vi "Periodic Tasks.vi"(8 "error in":errorcluster, 11 "RobotConfig":T6={"Motors"={"RightDrivePrimary"={"CAN Address"=0, "Invert"=FALSE, "InvertSensor"=FALSE, "Unit Conversion Factor"=0.0, "Brake Mode"=enum."Override to Brake", "Reverse Limt Switch Mode"=enum."Disabled", "Forward Limt Swith Mode"=enum."Disabled", "PWM Channel"=enum."Invalid", "Motor Controller Type"=enum."Talon SRX", "Peak Current (A)"=0, "Continuous Current (A)"=0, "Peak Duration (ms)"=0, "Current Limit Enable"=FALSE}, "RightDriveSecondary"={"CAN Address"=0, "Invert"=FALSE, "InvertSensor"=FALSE, "Unit Conversion Factor"=0.0, "Brake Mode"=enum."Override to Brake", "Reverse Limt Switch Mode"=enum."Disabled", "Forward Limt Swith Mode"=enum."Disabled", "PWM Channel"=enum."Invalid", "Motor Controller Type"=enum."Talon SRX", "Peak Current (A)"=0, "Continuous Current (A)"=0, "Peak Duration (ms)"=0, "Current Limit Enable"=FALSE}, "LeftDrivePrimary"={"CAN Address"=0, "Invert"=FALSE, "InvertSensor"=FALSE, "Unit Conversion Factor"=0.0, "Brake Mode"=enum."Override to Brake", "Reverse Limt Switch Mode"=enum."Disabled", "Forward Limt Swith Mode"=enum."Disabled", "PWM Channel"=enum."Invalid", "Motor Controller Type"=enum."Talon SRX", "Peak Current (A)"=0, "Continuous Current (A)"=0, "Peak Duration (ms)"=0, "Current Limit Enable"=FALSE}, "LeftDriveSecondary"={"CAN Address"=0, "Invert"=FALSE, "InvertSensor"=FALSE, "Unit Conversion Factor"=0.0, "Brake Mode"=enum."Override to Brake", "Reverse Limt Switch Mode"=enum."Disabled", "Forward Limt Swith Mode"=enum."Disabled", "PWM Channel"=enum."Invalid", "Motor Controller Type"=enum."Talon SRX", "Peak Current (A)"=0, "Continuous Current (A)"=0, "Peak Duration (ms)"=0, "Current Limit Enable"=FALSE}, "RightShooter"={"CAN Address"=0, "Invert"=FALSE, "InvertSensor"=FALSE, "Unit Conversion Factor"=0.0, "Brake Mode"=enum."Override to Brake", "Reverse Limt Switch Mode"=enum."Disabled", "Forward Limt Swith Mode"=enum."Disabled", "PWM Channel"=enum."Invalid", "Motor Controller Type"=enum."Talon SRX", "Peak Current (A)"=0, "Continuous Current (A)"=0, "Peak Duration (ms)"=0, "Current Limit Enable"=FALSE}, "LeftShooter"={"CAN Address"=0, "Invert"=FALSE, "InvertSensor"=FALSE, "Unit Conversion Factor"=0.0, "Brake Mode"=enum."Override to Brake", "Reverse Limt Switch Mode"=enum."Disabled", "Forward Limt Swith Mode"=enum."Disabled", "PWM Channel"=enum."Invalid", "Motor Controller Type"=enum."Talon SRX", "Peak Current (A)"=0, "Continuous Current (A)"=0, "Peak Duration (ms)"=0, "Current Limit Enable"=FALSE}, "ShooterRotate"={"CAN Address"=0, "Invert"=FALSE, "InvertSensor"=FALSE, "Unit Conversion Factor"=0.0, "Brake Mode"=enum."Override to Brake", "Reverse Limt Switch Mode"=enum."Disabled", "Forward Limt Swith Mode"=enum."Disabled", "PWM Channel"=enum."Invalid", "Motor Controller Type"=enum."Talon SRX", "Peak Current (A)"=0, "Continuous Current (A)"=0, "Peak Duration (ms)"=0, "Current Limit Enable"=FALSE}, "ShooterHood"={"CAN Address"=0, "Invert"=FALSE, "InvertSensor"=FALSE, "Unit Conversion Factor"=0.0, "Brake Mode"=enum."Override to Brake", "Reverse Limt Switch Mode"=enum."Disabled", "Forward Limt Swith Mode"=enum."Disabled", "PWM Channel"=enum."Invalid", "Motor Controller Type"=enum."Talon SRX", "Peak Current (A)"=0, "Continuous Current (A)"=0, "Peak Duration (ms)"=0, "Current Limit Enable"=FALSE}, "HopperWheel"={"CAN Address"=0, "Invert"=FALSE, "InvertSensor"=FALSE, "Unit Conversion Factor"=0.0, "Brake Mode"=enum."Override to Brake", "Reverse Limt Switch Mode"=enum."Disabled", "Forward Limt Swith Mode"=enum."Disabled", "PWM Channel"=enum."Invalid", "Motor Controller Type"=enum."Talon SRX", "Peak Current (A)"=0, "Continuous Current (A)"=0, "Peak Duration (ms)"=0, "Current Limit Enable"=FALSE}, "Elevator"={"CAN Address"=0, "Invert"=FALSE, "InvertSensor"=FALSE, "Unit Conversion Factor"=0.0, "Brake Mode"=enum."Override to Brake", "Reverse Limt Switch Mode"=enum."Disabled", "Forward Limt Swith Mode"=enum."Disabled", "PWM Channel"=enum."Invalid", "Motor Controller Type"=enum."Talon SRX", "Peak Current (A)"=0, "Continuous Current (A)"=0, "Peak Duration (ms)"=0, "Current Limit Enable"=FALSE}, "ClimberLeft"={"CAN Address"=0, "Invert"=FALSE, "InvertSensor"=FALSE, "Unit Conversion Factor"=0.0, "Brake Mode"=enum."Override to Brake", "Reverse Limt Switch Mode"=enum."Disabled", "Forward Limt Swith Mode"=enum."Disabled", "PWM Channel"=enum."Invalid", "Motor Controller Type"=enum."Talon SRX", "Peak Current (A)"=0, "Continuous Current (A)"=0, "Peak Duration (ms)"=0, "Current Limit Enable"=FALSE}, "ClimberRight"={"CAN Address"=0, "Invert"=FALSE, "InvertSensor"=FALSE, "Unit Conversion Factor"=0.0, "Brake Mode"=enum."Override to Brake", "Reverse Limt Switch Mode"=enum."Disabled", "Forward Limt Swith Mode"=enum."Disabled", "PWM Channel"=enum."Invalid", "Motor Controller Type"=enum."Talon SRX", "Peak Current (A)"=0, "Continuous Current (A)"=0, "Peak Duration (ms)"=0, "Current Limit Enable"=FALSE}, "Intake"={"CAN Address"=0, "Invert"=FALSE, "InvertSensor"=FALSE, "Unit Conversion Factor"=0.0, "Brake Mode"=enum."Override to Brake", "Reverse Limt Switch Mode"=enum."Disabled", "Forward Limt Swith Mode"=enum."Disabled", "PWM Channel"=enum."Invalid", "Motor Controller Type"=enum."Talon SRX", "Peak Current (A)"=0, "Continuous Current (A)"=0, "Peak Duration (ms)"=0, "Current Limit Enable"=FALSE}, "ControlPanel"={"CAN Address"=0, "Invert"=FALSE, "InvertSensor"=FALSE, "Unit Conversion Factor"=0.0, "Brake Mode"=enum."Override to Brake", "Reverse Limt Switch Mode"=enum."Disabled", "Forward Limt Swith Mode"=enum."Disabled", "PWM Channel"=enum."Invalid", "Motor Controller Type"=enum."Talon SRX", "Peak Current (A)"=0, "Continuous Current (A)"=0, "Peak Duration (ms)"=0, "Current Limit Enable"=FALSE}}, "PID"={"Shooter"={"P"=0.0, "I"=0.0, "D"=0.0, "F"=0.0, "IZone"=0.0}, "Turret"={"P"=0.0, "I"=0.0, "D"=0.0, "F"=0.0, "IZone"=0.0}, "Elevator"={"P"=0.0, "I"=0.0, "D"=0.0, "F"=0.0, "IZone"=0.0}, "ControlPanel"={"P"=0.0, "I"=0.0, "D"=0.0, "F"=0.0, "IZone"=0.0}, "Hood"={"P"=0.0, "I"=0.0, "D"=0.0, "F"=0.0, "IZone"=0.0}}, "MotionMagic"={"Turret"={"CruiseVelocity"=0, "Acceleration"=0}, "Elevator"={"CruiseVelocity"=0, "Acceleration"=0}, "ControlPanel"={"CruiseVelocity"=0, "Acceleration"=0}}, "Sensors"={"IMU"={"Yaw Axis"=enum."Z", "SPI Bus"=enum."SPI MXP", "AHRS Algorithm"=enum."Complementary", "Calibration Time (s)"=3.0, "Calibrate On Open"=TRUE}, "ElevatorBottom"={"ID"=0, "RangingMode"=enum."Short", "sampleTime(ms)"=24.0}, "ElevatorTop"={"ID"=0, "RangingMode"=enum."Short", "sampleTime(ms)"=24.0}, "ControlPanelColorSensor"={"alsIntegrationTime(ms)"=10.0, "alsGain"=40, "I2C Bus"=enum."I2C On-Board", "numProximityPulses"=5, "proximityGain"=1, "proximityLEDCurrent(mA)"=50, "proximityPulseLength(ms)"=0.01, "proximitySampleTime(ms)"=10.0}}, "Solenoids"={"Intake"={"SolenoidChannel"=enum."Solenoid 0", "Invert"=FALSE}, "ClimberRachet"={"SolenoidChannel"=enum."Solenoid 0", "Invert"=FALSE}}, "EnableCompressor"=FALSE, "RobotDimensions"={"Wheelbase(in)"=0.0, "Length(in)"=0.0}, "CameraMounting"={"LensHeight(in)"=0.0, "RotationRadius(in)"=0.0, "Pitch(deg)"=0.0}, "SensorCalibrations"={"TopToFMinBallDistance(in)"=0.0, "BottomToFMinBallDistance(in)"=0.0}, "Homing"={"Hood Homing Position (deg)"=0.0, "Turret Homing Position (deg)"=0.0}, "MotionLimits"={"Hood"={"Min (deg)"=0.0, "Max (deg)"=0.0}, "Turret"={"Min (deg)"=0.0, "Max (deg)"=0.0}}} {"Sensors"."ElevatorTop"."sampleTime(ms)" min=24.0 max=1000.0 step=1.0; "Sensors"."ElevatorBottom"."sampleTime(ms)" min=24.0 max=1000.0 step=1.0}) -> ()   [LabVIEW 2019]
doc: "This VI runs in parallel to other tasks. It can contain as many user-defined periodic loops as you need. These can carry out PID or other sorts of timed response."
uses:
  ArgosLib/ArgosLib.lvlib
  InfiniteRechargeSrc/Global_Var-RefNum/JoystickControls.vi
  InfiniteRechargeSrc/Implements/Shooter/TypeDefs/Hood_Homing_State.ctl
  InfiniteRechargeSrc/Vision/TypeDefs/VisionPipeline.ctl
  <vilib>/Playing With Fusion Inc/Playing With Fusion Lib for FRC/PWF_TMD37003_LabVIEW/PwF_TMD37003.lvlib
  <vilib>/Playing With Fusion Inc/Playing With Fusion Lib for FRC/PWF_TMD37003_LabVIEW/Public/PwF_TMD37003_RGBToHSV_SensorData.vi
  <vilib>/Rock Robotics/WPI/ThirdParty/Phoenix-LabVIEW/Motor Controller/Controls/CTRE_Phoenix_MotorControl_NeutralMode.ctl
  <vilib>/Rock Robotics/WPI/ThirdParty/Phoenix-LabVIEW/Motor Controller/Controls/CTRE_Phoenix_MotorControl_LimitSwitchNormal.ctl
  <vilib>/Rock Robotics/SystemInterfaces/DIO/FPGA_DIOPWMChannel.ctl
  ArgosLib/Config/ConfigComponents/TypeDefs/Config_MotorCtrlType.ctl
  ArgosLib/Config/ConfigComponents/TypeDefs/Config_Motor.ctl
  ArgosLib/Config/ConfigComponents/TypeDefs/Config_PIDParams.ctl
  ArgosLib/Config/ConfigComponents/TypeDefs/Config_MotionMagicParams.ctl
  <vilib>/Rock Robotics/SystemInterfaces/spilib/spi_bus.ctl
  ArgosLib/Config/ConfigComponents/TypeDefs/Config_IMU.ctl
  <vilib>/Rock Robotics/WPI/Solenoid/WPI_SolenoidChannel.ctl
  ArgosLib/Config/ConfigComponents/TypeDefs/Config_SingleSolenoid.ctl
  InfiniteRechargeSrc/TypeDefs/ConfigComponents/Config_RobotDimensions.ctl
  InfiniteRechargeSrc/TypeDefs/ConfigComponents/Config_CameraMounting.ctl
  InfiniteRechargeSrc/TypeDefs/ConfigComponents/Config_Robot.ctl
  <vilib>/Playing With Fusion Inc/Playing With Fusion Lib for FRC/PWF_ToF_LabVIEW/Public/TypeDefs/PwF_ToF_RangingMode.ctl
  <vilib>/Playing With Fusion Inc/Playing With Fusion Lib for FRC/PWF_ToF_LabVIEW/PwF_ToF.lvlib
  ArgosLib/Config/ConfigComponents/TypeDefs/Config_PwFToF.ctl
  ArgosLib/Miscellaneous/TypeDefs/LookUpTableParameters.ctl
  ArgosLib/Miscellaneous/TypeDefs/ArgoDriveJoystickMap.ctl
  InfiniteRechargeSrc/Implements/Control_Panel/TypeDefs/ControlPanelColor.ctl
  <vilib>/Playing With Fusion Inc/Playing With Fusion Lib for FRC/PWF_TMD37003_LabVIEW/Public/TypeDefs/PwF_TMD37003_Data.ctl
  <vilib>/Rock Robotics/SystemInterfaces/i2clib/i2c_bus.ctl
  ArgosLib/Config/ConfigComponents/TypeDefs/Config_PwF_TMD37003.ctl
panel:
  out "TMD37003 Data":T1
  out "Color":T2=enum."Blue"
  out "Turret Distance (in)":dbl
  out "Shooter Velocity":dbl
  in  "ManualShooterSpeed":bool
  in  "ShooterSpeed(rpm)":dbl(slide)=4000.0 min=0.0 max=10000.0 step=1.0 scale=0.0..10000.0
  in  "DisableLimelight":bool
  out "Target Found?":bool
  in  "SetPointTurret(Deg)":dbl(slide) scale=-108.0..108.0
  in  "Activate Auto (Turret)":bool
  out "TurretManual":bool
  out "Turret Current Position (Deg)":dbl
  out "Hood Current Position (Deg)":dbl
  out "HoodManual?":bool
  in  "Activate Auto (Shooter Hood)":bool
  in  "SetPointHood(Deg)":dbl
  in  "TurretHomeReset":bool
  in  "Turret Homing Activated":bool
  out "Turret Homing_State":T3
  in  "HoodHomeActivate":bool
  in  "HoodHomeReset":bool
  out "Hood_Homing_State":T3
  in  "Argo Drive Joystick Map":T4={"Auto Speed"={"Look Up Table OUT"=[-1.0, 0.0, 1.0], "Look Up Table IN"=[-1.0, 0.0, 1.0]}, "Low Speed"={"Look Up Table OUT"=[-1.0, 0.0, 0.0, 1.0], "Look Up Table IN"=[-1.0, -0.25, 0.25, 1.0]}, "Auto Turning"={"Look Up Table OUT"=[-1.0, 0.0, 1.0], "Look Up Table IN"=[-1.0, 0.0, 1.0]}, "Low Turning"={"Look Up Table OUT"=[-1.0, 0.0, 0.0, 1.0], "Look Up Table IN"=[-1.0, -0.25, 0.25, 1.0]}, "High Speed"={"Look Up Table OUT"=[], "Look Up Table IN"=[]}, "High Turning"={"Look Up Table OUT"=[], "Look Up Table IN"=[]}}
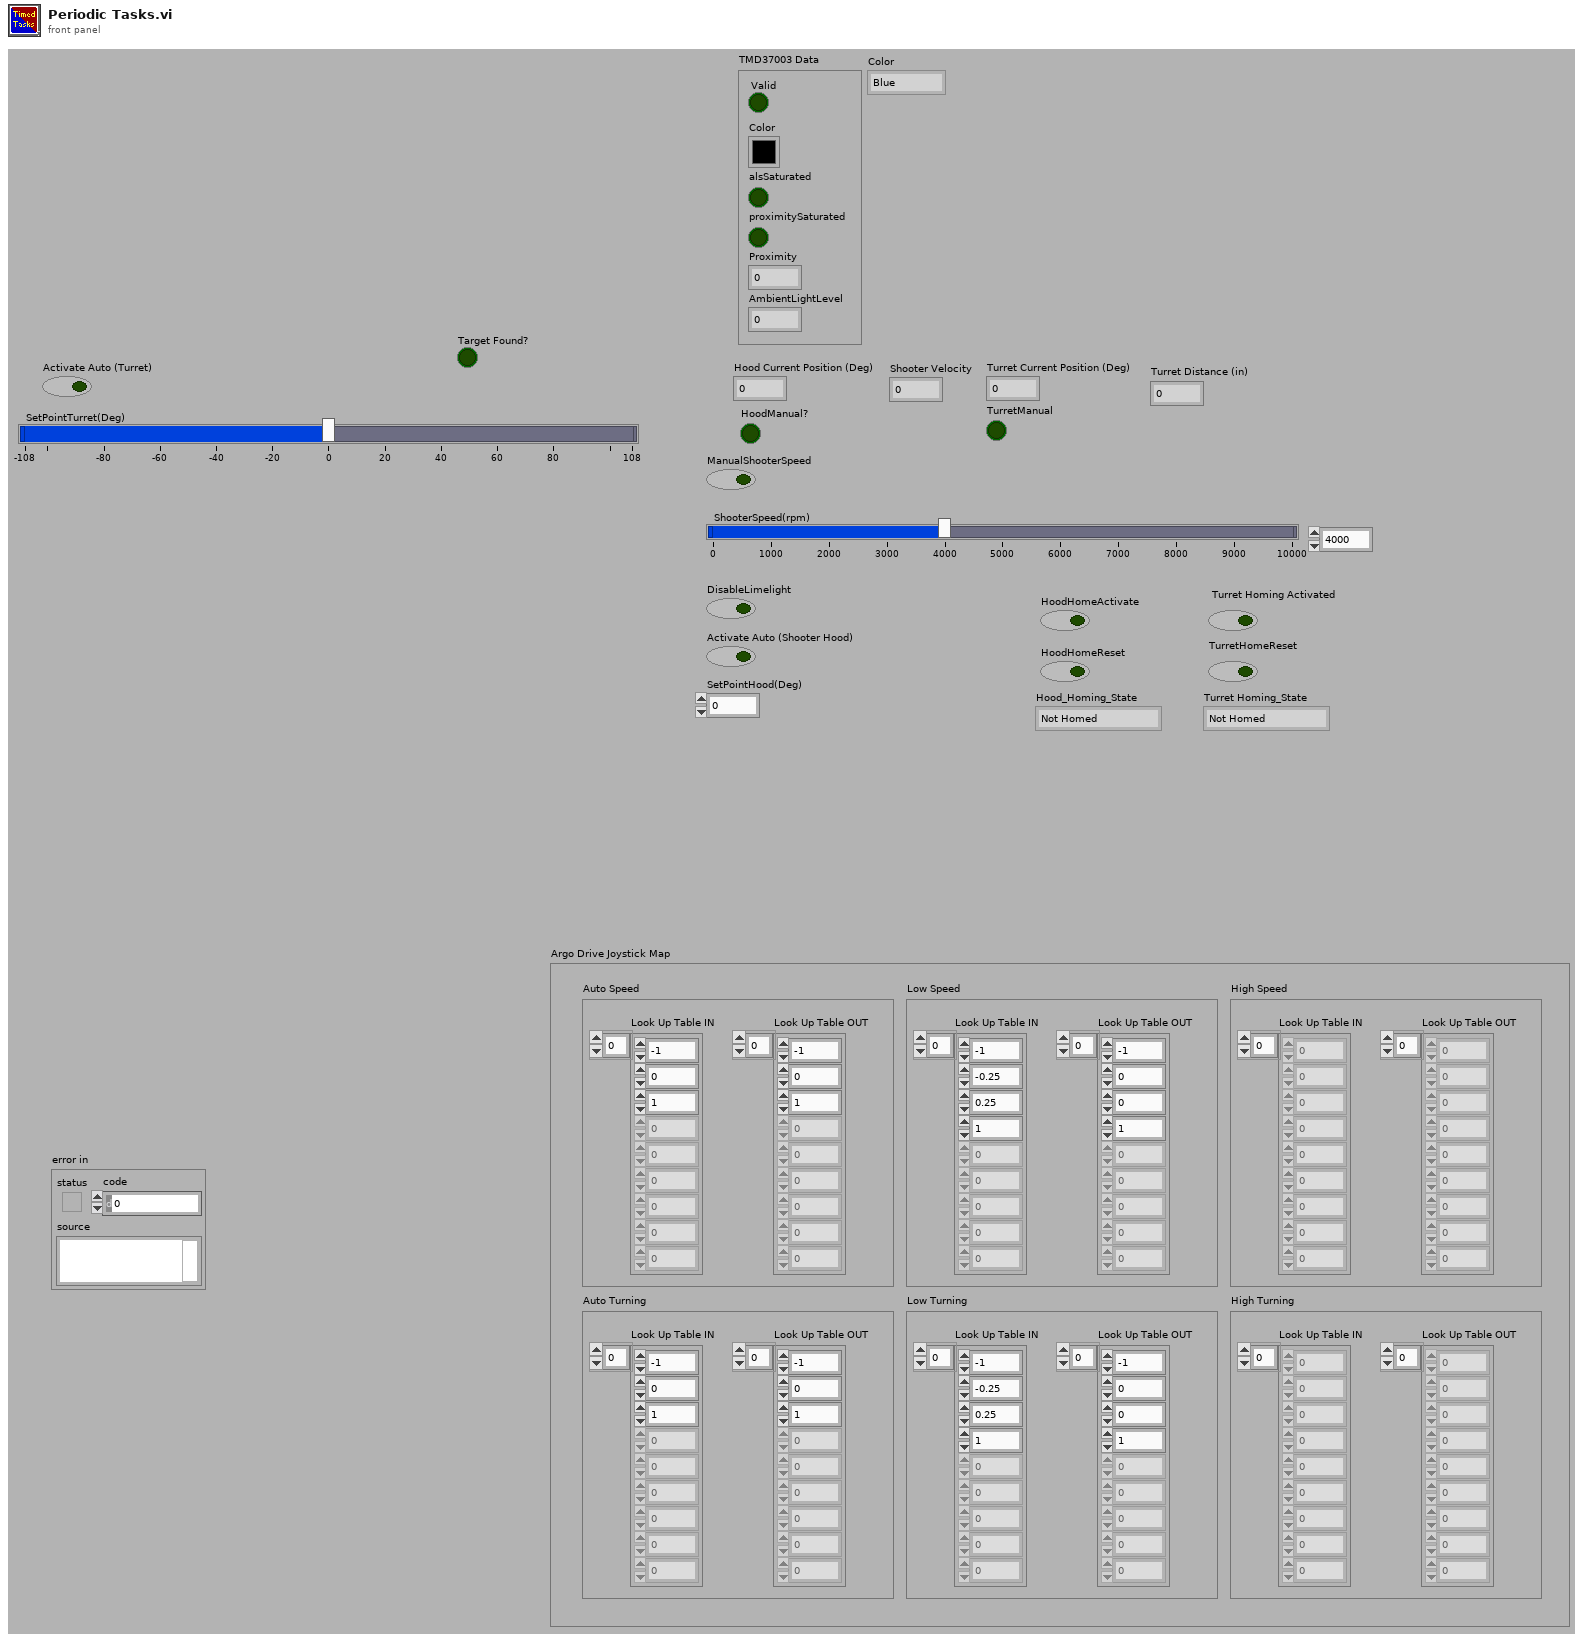
[diagram p1: front panel]
types:
  T1 = typedef "PlayingWithFusionLib.lvlib/PwF_TMD37003.lvlib/PwF_TMD37003_Data.ctl" = cluster{"Valid":bool, "Color":u32, "alsSaturated":bool, "proximitySaturated":bool, "Proximity":dbl, "AmbientLightLevel":dbl}
  T2 = typedef "ControlPanelColor.ctl" = enum16{"Unknown", "Red", "Green", "Blue", "Yellow"}
  T3 = typedef "Hood_Homing_State.ctl" = enum16{"Not Homed", "Homing in Process", "Homing Failed", "Homing Completed"}
  T4 = typedef "ArgosLib.lvlib/ArgoDriveJoystickMap.ctl" = cluster{"Auto Speed":T5, "Low Speed":T5, "Auto Turning":T5, "Low Turning":T5, "High Speed":T5, "High Turning":T5}
  T5 = typedef "ArgosLib.lvlib/LookUpTableParameters.ctl" = cluster{"Look Up Table OUT":dbl[], "Look Up Table IN":dbl[]}
  T6 = typedef "Config_Robot.ctl" = cluster{"Motors":cluster{"RightDrivePrimary":T7, "RightDriveSecondary":T7, "LeftDrivePrimary":T7, "LeftDriveSecondary":T7, "RightShooter":T7, "LeftShooter":T7, "ShooterRotate":T7, "ShooterHood":T7, "HopperWheel":T7, "Elevator":T7, "ClimberLeft":T7, "ClimberRight":T7, "Intake":T7, "ControlPanel":T7}, "PID":cluster{"Shooter":T12, "Turret":T12, "Elevator":T12, "ControlPanel":T12, "Hood":T12}, "MotionMagic":cluster{"Turret":T13, "Elevator":T13, "ControlPanel":T13}, "Sensors":cluster{"IMU":T14, "ElevatorBottom":T16, "ElevatorTop":T16, "ControlPanelColorSensor":T18}, "Solenoids":cluster{"Intake":T20, "ClimberRachet":T20}, "EnableCompressor":bool, "RobotDimensions":T22, "CameraMounting":T23, "SensorCalibrations":cluster{"TopToFMinBallDistance(in)":dbl, "BottomToFMinBallDistance(in)":dbl}, "Homing":cluster{"Hood Homing Position (deg)":dbl, "Turret Homing Position (deg)":dbl}, "MotionLimits":cluster{"Hood":cluster{"Min (deg)":dbl, "Max (deg)":dbl}, "Turret":cluster{"Min (deg)":dbl, "Max (deg)":dbl}}}
  T7 = typedef "ArgosLib.lvlib/Config_Motor.ctl" = cluster{"CAN Address":u8, "Invert":bool, "InvertSensor":bool, "Unit Conversion Factor":dbl, "Brake Mode":T8, "Reverse Limt Switch Mode":T9, "Forward Limt Swith Mode":T9, "PWM Channel":T10, "Motor Controller Type":T11, "Peak Current (A)":i32, "Continuous Current (A)":i32, "Peak Duration (ms)":i32, "Current Limit Enable":bool}
  T8 = typedef "CTRE_Phoenix_MotorControl_NeutralMode.ctl" = enum8{"EEPROMSetting", "Override to Coast", "Override to Brake"}
  T9 = typedef "CTRE_Phoenix_MotorControl_LimitSwitchNormal.ctl" = enum16{"Normally Open", "Normally Closed", "Disabled"}
  T10 = typedef "FPGA_DIOPWMChannel.ctl" = enum8{"PWM 0", "PWM 1", "PWM 2", "PWM 3", "PWM 4", "PWM 5", "PWM 6", "PWM 7", "PWM 8", "PWM 9", "PWM MXP 0", "PWM MXP 1", "PWM MXP 2", "PWM MXP 3", "PWM MXP 4", "PWM MXP 5", "PWM MXP 6", "PWM MXP 7", "PWM MXP 8", "PWM MXP 9", "Invalid"}
  T11 = typedef "ArgosLib.lvlib/Config_MotorCtrlType.ctl" = enum16{"Disabled", "Talon SRX", "Talon SR", "Venom", "Spark MAX", "Falcon FX"}
  T12 = typedef "ArgosLib.lvlib/Config_PIDParams.ctl" = cluster{"P":dbl, "I":dbl, "D":dbl, "F":dbl, "IZone":dbl}
  T13 = typedef "ArgosLib.lvlib/Config_MotionMagicParams.ctl" = cluster{"CruiseVelocity":i32, "Acceleration":i32}
  T14 = typedef "ArgosLib.lvlib/Config_IMU.ctl" = cluster{"Yaw Axis":enum16{"X", "Y", "Z"}, "SPI Bus":T15, "AHRS Algorithm":enum16{"Complementary", "Madgwick"}, "Calibration Time (s)":dbl, "Calibrate On Open":bool}
  T15 = typedef "spi_bus.ctl" = enum16{"SPI On-Board, CS0", "SPI On-Board, CS1", "SPI On-Board, CS2", "SPI On-Board, CS3", "SPI MXP", "Invalid"}
  T16 = typedef "ArgosLib.lvlib/Config_PwFToF.ctl" = cluster{"ID":u8, "RangingMode":T17, "sampleTime(ms)":dbl}
  T17 = typedef "PlayingWithFusionLib.lvlib/PwF_ToF.lvlib/PwF_ToF_RangingMode.ctl" = enum16{"Short", "Medium", "Long"}
  T18 = typedef "ArgosLib.lvlib/Config_PwF_TMD37003.ctl" = cluster{"alsIntegrationTime(ms)":dbl, "alsGain":u8, "I2C Bus":T19, "numProximityPulses":u8, "proximityGain":u8, "proximityLEDCurrent(mA)":u8, "proximityPulseLength(ms)":dbl, "proximitySampleTime(ms)":dbl}
  T19 = typedef "i2c_bus.ctl" = enum16{"I2C On-Board", "I2C MXP", "Invalid"}
  T20 = typedef "ArgosLib.lvlib/Config_SingleSolenoid.ctl" = cluster{"SolenoidChannel":T21, "Invert":bool}
  T21 = typedef "WPI_SolenoidChannel.ctl" = enum8{"Solenoid 0", "Solenoid 1", "Solenoid 2", "Solenoid 3", "Solenoid 4", "Solenoid 5", "Solenoid 6", "Solenoid 7", "Invalid"}
  T22 = typedef "Config_RobotDimensions.ctl" = cluster{"Wheelbase(in)":dbl, "Length(in)":dbl}
  T23 = typedef "Config_CameraMounting.ctl" = cluster{"LensHeight(in)":dbl, "RotationRadius(in)":dbl, "Pitch(deg)":dbl}
  T24 = typedef "SensorRefNums.ctl" = cluster{"ElevatorBottom":T25, "ElevatorTop":T25, "ControlPanelColor":T26}
  T25 = typedef "PlayingWithFusionLib.lvlib/PwF_ToF.lvlib/PwF_ToF_DevRef.ctl" = cluster{"DeviceStatus":errorcluster, "Device Number":u8, "Handle":u64, "Library Path":path}
  T26 = typedef "PlayingWithFusionLib.lvlib/PwF_TMD37003.lvlib/PwF_TMD37003_DevRef.ctl" = cluster{"DevStatus":errorcluster, "Device Address":u8, "Handle":i32, "I2C Bus":T19}
  T27 = typedef "JoystickRefNums.ctl" = cluster{"Joystick0":T28, "Joystick1":T28}
  T28 = typedef "WPI_JoystickDevRef.ctl" = cluster{"Device":T29}
  T29 = typedef "WPI_JoystickDeviceEnum.ctl" = enum16{"USB 0", "USB 1", "USB 2", "USB 3", "USB 4", "USB 5"}
  T30 = typedef "WPI_RobotDriveDevRef.ctl" = cluster{"DevStatus":errorcluster, "Motors[]":T31[], "Square Inputs":bool, "Max Output":dbl}
  T31 = typedef "WPI_MotorControlDeviceRef.ctl" = cluster{"DeviceStatus":errorcluster, "Type":T32, "PWM":cluster{"PWM Channel":T10, "DeadBand":T33}, "CAN":cluster{"Device Number":u8, "SetOutput VI Ref":variant, "GetOutput VI Ref":variant, "Enable VI Ref":variant, "Disable VI Ref":variant, "Data":variant}, "Invert":bool, "DIO PWM":cluster{"PWM \"Enable\" Channel":T10, "DIOChannel":T34, "PWM Rate":dbl}}
  T32 = typedef "WPI_MotorControlType.ctl" = enum16{"PWM", "CAN", "DIO PWM"}
  T33 = typedef "WPI_PWMDeadband.ctl" = cluster{"Name":string, "maxPositivePwm":i32, "minPositivePwm":i32, "centerPwm":i32, "maxNegativePwm":i32, "minNegativePwm":i32, "angularRange":u16}
  T34 = typedef "FPGA_DIOChannel.ctl" = enum8{"DIO 0", "DIO 1", "DIO 2", "DIO 3", "DIO 4", "DIO 5", "DIO 6", "DIO 7", "DIO 8", "DIO 9", "DIO MXP 0", "DIO MXP 1", "DIO MXP 2", "DIO MXP 3", "DIO MXP 4", "DIO MXP 5", "DIO MXP 6", "DIO MXP 7", "DIO MXP 8", "DIO MXP 9", "DIO MXP 10", "DIO MXP 11", "DIO MXP 12", "DIO MXP 13", "DIO MXP 14", "DIO MXP 15", "SPI Port CS1", "SPI Port CS2", "SPI Port CS3", "SPI Port MISO", "SPI Port MOSI", "Invalid"}
  T35 = typedef "PneumaticsRefNums.ctl" = cluster{"Intake":T36, "Compressor":T37, "ClimberRatchet":T36}
  T36 = typedef "WPI_SolenoidDevRef.ctl" = cluster{"DevStatus":errorcluster, "Pneumatics Control Module":u8, "Forward Solenoid Channel":T21, "Reverse Solenoid Channel":T21}
  T37 = typedef "WPI_CompressorDevRef.ctl" = cluster{"DevStatus":errorcluster, "Pneumatics Control Module":u8}
  T38 = typedef "MotorRefNums.ctl" = cluster{"LeftDrivePrimary":T31, "RightDrivePrimary":T31, "LeftDriveSecondary":T31, "RightDriveSecondary":T31, "RightShooter":T31, "LeftShooter":T31, "ShooterRotate":T31, "ShooterHood":T31, "HopperWheel":T31, "Elevator":T31, "ClimberLeft":T31, "ClimberRight":T31, "Intake":T31, "ControlPanel":T31}
  T39 = cluster{"RobotConfig":T6, "JoystickRefNums":T27, "RobotDriveDevRef":T30, "MotorRefNumsOut":T38, "Pneumatics":T35, "Sensors":T24}
  T40 = typedef "JoystickControl.ctl" = cluster{"A":bool, "B":bool, "X":bool, "Y":bool, "LB":bool, "Shoot":bool, "LJ":bool, "RJ":bool, "Back":bool, "Start":bool, "Top":bool, "Right":bool, "Bottom":bool, "Left":bool, "Eject":dbl, "Intake":dbl, "LX":dbl, "Drive Y":dbl, "Drive X":dbl, "RY":dbl, "Down":bool, "Index":bool, "Aggitate":bool, "Up":bool, "Find Target":bool, "Spin up":bool, "LJ 2":bool, "RJ 2":bool, "Back 2":bool, "Start 2":bool, "Elevate":bool, "Right 2":bool, "Retract":bool, "Left 2":bool, "Control Rotate":dbl, "RT 2":dbl, "H L/R":dbl, "H U/D":dbl, "RX 2":dbl, "RY 2":dbl}
  T41 = typedef "VisionPipeline.ctl" = enum16{"LEDOff", "NoZoom", "Zoom2x", "Zoom3x"}
  T42 = typedef "VisionTarget.ctl" = cluster{"Valid":bool, "Distance(in)":dbl, "Angle(deg)":dbl, "FieldCentricAngle(deg)":dbl, "skew (deg)":dbl}
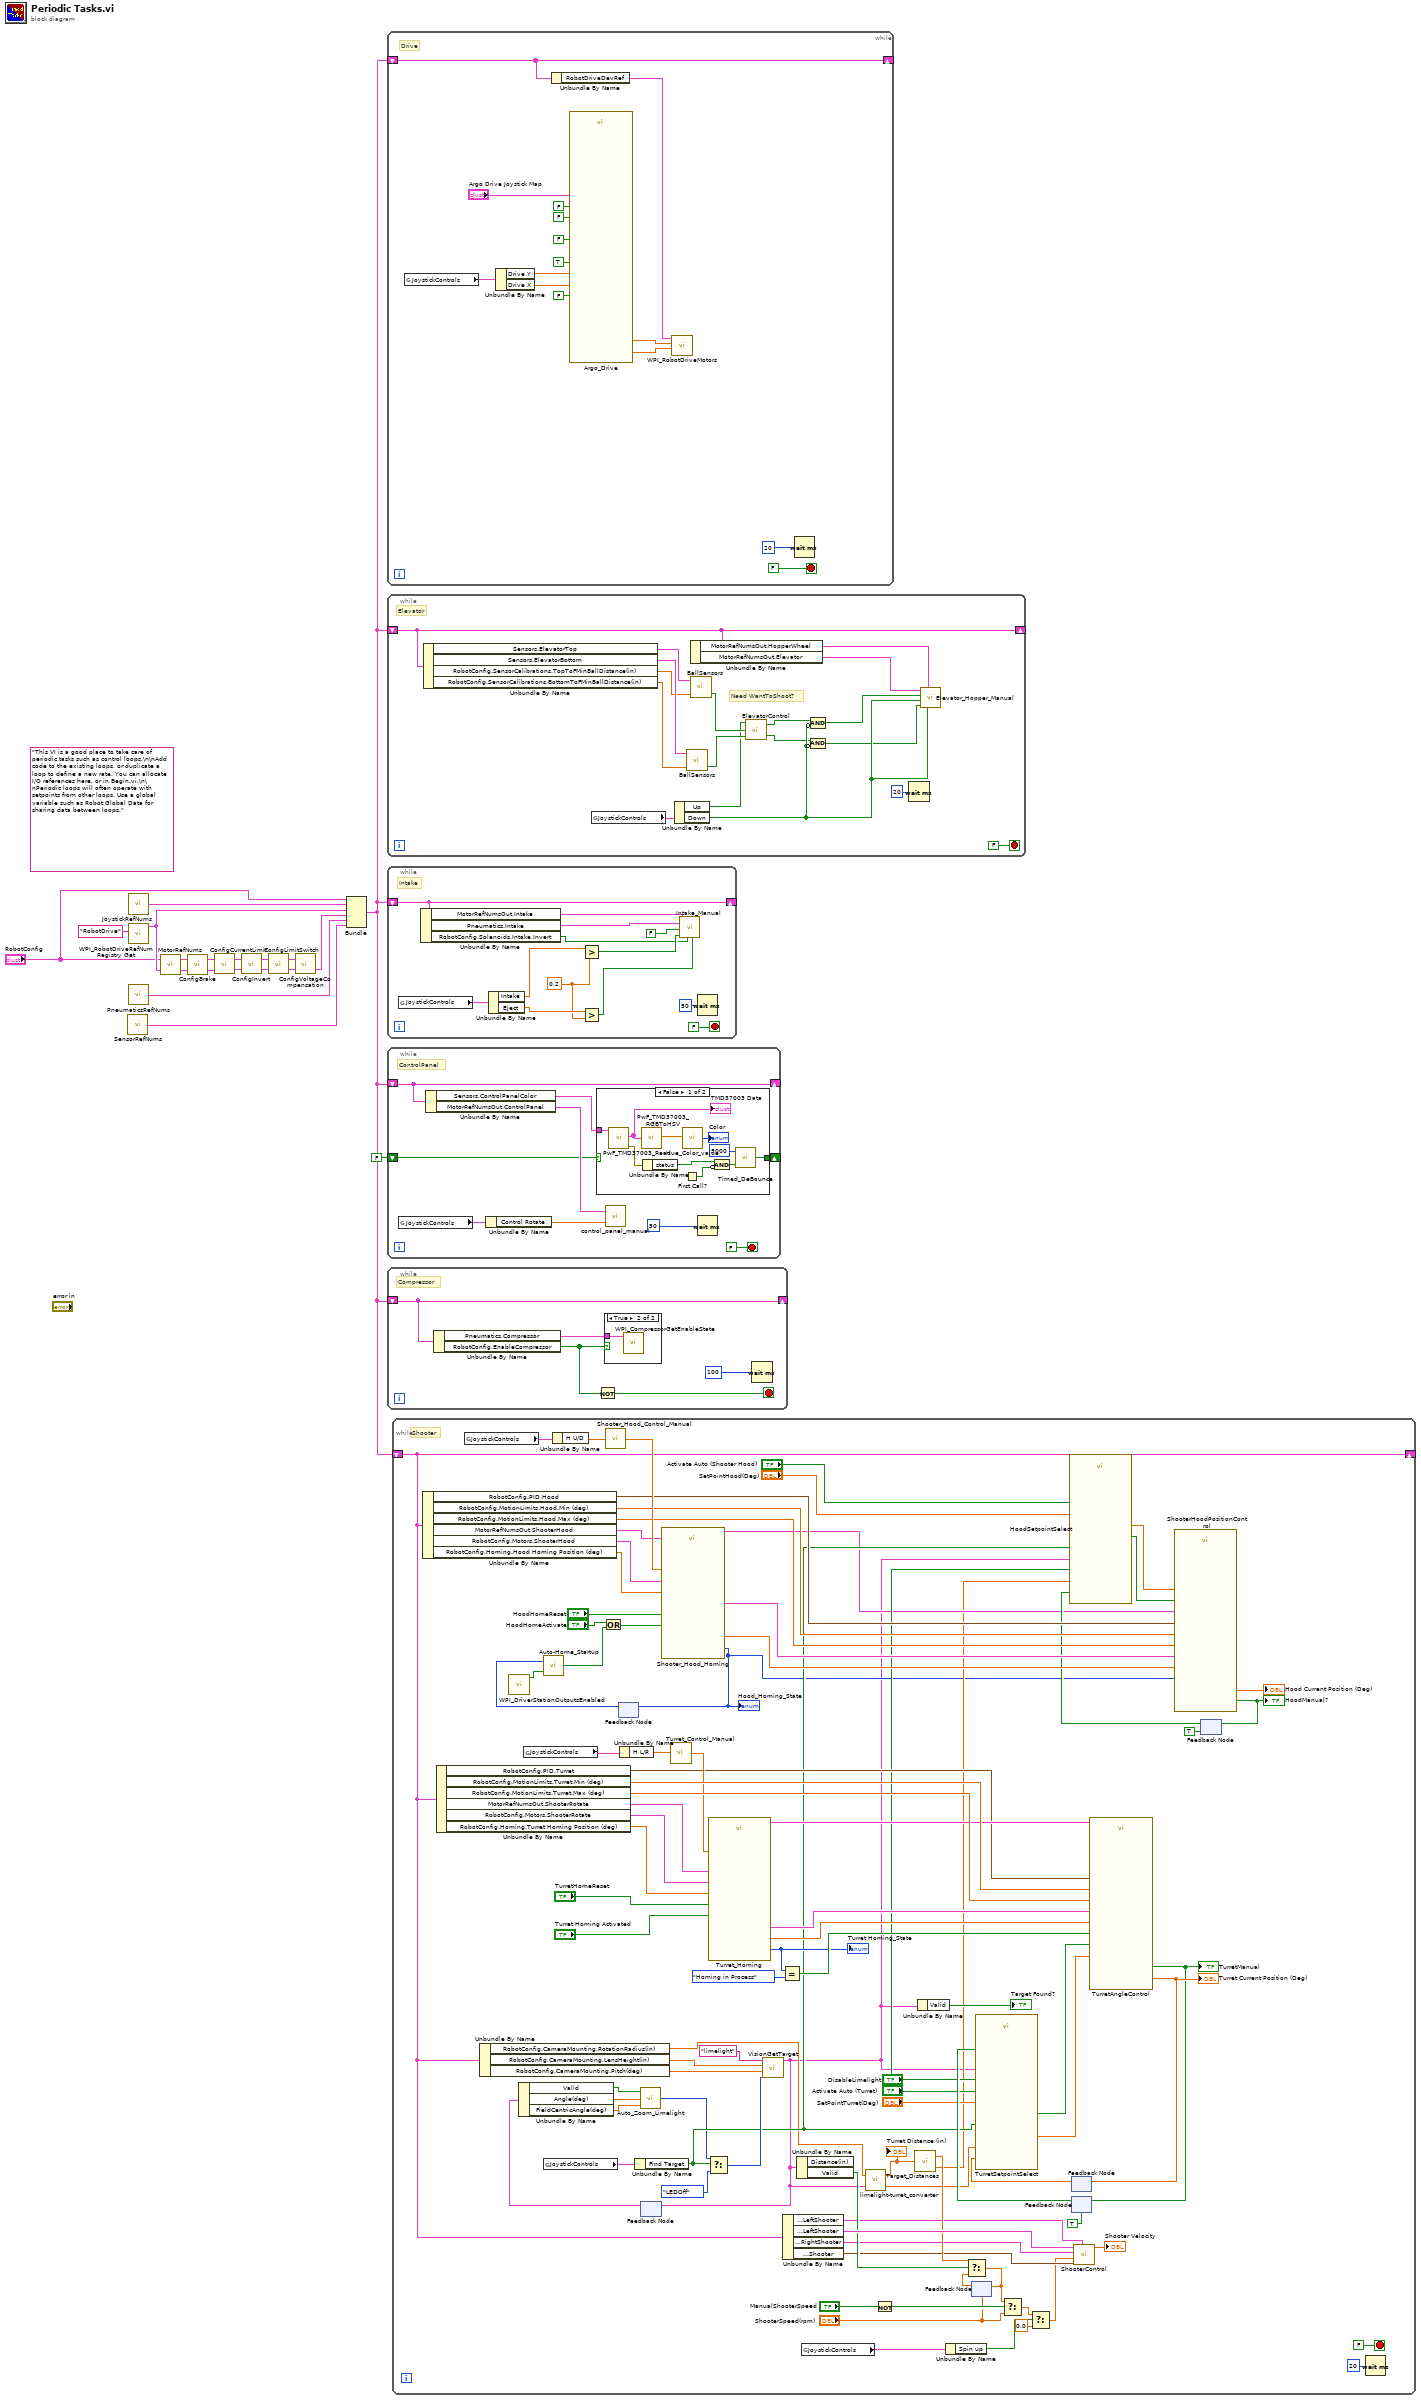
[diagram p0: block diagram]
diagram:
  (unwired) "This VI is a good place to take care of periodic tasks such as control loops.\n\nAdd code to the existing loops, or duplicate a loop to define a new rate. You can allocate I/O references here, or in Begin.vi.\n\nPeriodic loops will often operate with setpoints from other loops. Use a global variable such as Robot Global Data for sharing data between loops."
  n1 = call "SensorRefNums.vi"() -> ("Sensors"=w15:T24)  [unwired: 1 in]
  n2 = call "JoystickRefNums.vi"() -> ("JoystickRefNums"=w19:T27)  [unwired: 1 in]
  n3 = call <vilib>:"WPI_RobotDriveRefNum Registry Get.vi"("refnum name"="RobotDrive") -> ("RobotDriveDevRef"=w17:T30)  [unwired: 9 in, 1 out]
  n4 = call "PneumaticsRefNums.vi"() -> ("Pneumatics"=w16:T35)  [unwired: 1 in]
  n5 = call "MotorRefNums.vi"("RobotDriveDevRef"=w17, "RobotConfig"="RobotConfig") -> ("MotorRefNums"=w13:T38, "RobotConfigOut"=w14:T6)
  n6 = call "ConfigBrake.vi"("MotorRefNumsIn"=w13, "RobotConfigIn"=w14) -> ("MotorRefNumsOut"=w12:T38, "RobotConfigOut"=w11:T6)
  n7 = call "ConfigCurrentLimit.vi"("MotorRefNumsIn"=w12, "RobotConfigIn"=w11) -> ("MotorRefNumsOut"=w10:T38, "RobotConfigOut"=w9:T6)
  n8 = call "ConfigInvert.vi"("MotorRefNumsIn"=w10, "RobotConfigIn"=w9) -> ("MotorRefNumsOut"=w8:T38, "RobotConfigOut"=w7:T6)
  n9 = call "ConfigLimitSwitch.vi"("MotorRefNumsIn"=w8, "RobotConfigIn"=w7) -> ("MotorRefNumsOut"=w6:T38, "RobotConfigOut"=w5:T6)
  n10 = call "ConfigVoltageCompensation.vi"("MotorRefNumsIn"=w6, "RobotConfigIn"=w5) -> ("MotorRefNumsOut"=w4:T38)  [unwired: 1 out]
  n11 = Bundle("RobotConfig"="RobotConfig", "JoystickRefNums"=w19, "RobotDriveDevRef"=w17, "MotorRefNumsOut"=w4, "Pneumatics"=w16, "Sensors"=w15) -> (w2:T39)  [unwired: 1 out]
  n12 = while {
    shift-right: [w32] -> _
    shift-left: w2 -> [w32]
    stop <- FALSE stop-if-true
    # "Drive"
    n13 = global read "JoystickControls.vi" "JoystickControls"() -> (w31:T40)
    n14 = Unbundle By Name(w31) -> ("Drive Y"=w30:dbl, "Drive X"=w29:dbl)
    n15 = Unbundle By Name(w32) -> ("RobotDriveDevRef"=w22:T30)
    n16 = call "Argo_Drive.vi"("Speed_Main"=w30, "Argo Drive Joystick Map"="Argo Drive Joystick Map", "Backwards_Turning_Flip"=FALSE, "Turning_PID_Enable"=FALSE, "Turning_Main"=w29, "Auto_Enable"=FALSE, "High_Gear"=FALSE, "Quick_Turn"=TRUE) -> ("Left_Motor"=w21:dbl, "Right_Motor"=w20:dbl)  [unwired: 10 in]
    n17 = call <vilib>:"WPI_RobotDriveMotors.vi"("RightSpeed"=w20, "LeftSpeed"=w21, "RobotDriveDevRef"=w22) -> ()  [unwired: 6 in, 3 out]
    n18 = Wait (ms)(milliseconds to wait=u32 20) -> ()  [unwired: 1 out]
  }
  n19 = while {
    shift-right: [w46] -> _
    shift-left: w2 -> [w46]
    stop <- FALSE stop-if-true
    # "Need WantToShoot?"
    # "Elevator"
    n20 = Unbundle By Name(w46) -> ("Sensors.ElevatorTop"=w48:T25, "Sensors.ElevatorBottom"=w47:T25, "RobotConfig.SensorCalibrations.TopToFMinBallDistance(in)"=w38:dbl, "RobotConfig.SensorCalibrations.BottomToFMinBallDistance(in)"=w37:dbl)
    n21 = global read "JoystickControls.vi" "JoystickControls"() -> (w45:T40)
    n22 = Unbundle By Name(w45) -> ("Up"=w39:bool, "Down"=w44:bool)
    n23 = call "BallSensors.vi"("MinDistance(in.)"=w37, "BallSensorDevRefIn"=w47) -> ("BallThere?"=w50:bool)  [unwired: 1 in, 2 out]
    n24 = Unbundle By Name(w46) -> ("MotorRefNumsOut.HopperWheel"=w35:T31, "MotorRefNumsOut.Elevator"=w36:T31)
    n25 = call "BallSensors.vi"("MinDistance(in.)"=w38, "BallSensorDevRefIn"=w48) -> ("BallThere?"=w49:bool)  [unwired: 1 in, 2 out]
    n26 = call "ElevatorControl.vi"("BallThereAtBottom?"=w50, "BallThereAtTop?"=w49, "WantToShoot?"=w39) -> ("HopperWheelsOn"=w42:bool, "ElevatorOn"=w43:bool)
    n27 = Compound Arithmetic op=AND(w43, invert w44) -> (w41:bool)
    n28 = Compound Arithmetic op=AND(w42, invert w44) -> (w40:bool)
    n29 = Wait (ms)(milliseconds to wait=u32 20) -> ()  [unwired: 1 out]
    n30 = call "Elevator_Hopper_Manual.vi"("Elevator_Control"=w36, "Hopper_Control"=w35, "Elevator_up"=w41, "Elevator_Down"=w44, "Hopper Backwards"=w44, "Hopper Forwards"=w40) -> ()  [unwired: 3 in]
  }
  n31 = while {
    shift-right: [w59] -> _
    shift-left: w2 -> [w59]
    stop <- FALSE stop-if-true
    w54 = 0.2 ("y")
    # "Intake"
    n32 = global read "JoystickControls.vi" "JoystickControls"() -> (w63:T40)
    n33 = Unbundle By Name(w59) -> ("MotorRefNumsOut.Intake"=w58:T31, "Pneumatics.Intake"=w57:T36, "RobotConfig.Solenoids.Intake.Invert"=w53:bool)
    n34 = Unbundle By Name(w63) -> ("Intake"=w56:dbl, "Eject"=w55:dbl)
    n35 = Greater?(x=w56, y=w54) -> (0:w60:bool)
    n36 = Greater?(x=w55, y=w54) -> (0:w61:bool)
    n37 = call "Intake_Manual.vi"("Reverse_Intake"=w61, "Invert Solenoid"=w53, "Intake"=w60, "Disable"=FALSE, "IntakeExtendDevRef"=w57, "Intake_Motor"=w58) -> ()  [unwired: 5 in]
    n38 = Wait (ms)(milliseconds to wait=u32 50) -> ()  [unwired: 1 out]
  }
  n39 = while {
    shift-right: [w72] -> _
    shift-left: w2 -> [w72]
    shift-right: [w68] -> _
    shift-left: FALSE ("Output") -> [w67]
    stop <- FALSE stop-if-true
    # "ControlPanel"
    n40 = global read "JoystickControls.vi" "JoystickControls"() -> (w73:T40)
    n41 = Unbundle By Name(w72) -> ("Sensors.ControlPanelColor"=w71:T26, "MotorRefNumsOut.ControlPanel"=w69:T31)
    n42 = Unbundle By Name(w73) -> ("Control Rotate"=w70:dbl)
    n43 = case shown="False" w67 {
      selector: w67 -> [_ w85]
      tunnel: w71 -> [w81 _]
      tunnel: [w78 w85] -> w68
      frame False {
        n44 = call <vilib>:"PwF_TMD37003_Read.vi"("PwF_TMD37003_DevRefIn"=w81) -> ("error out"=w80:errorcluster, "TMD37003 Data"=w84:T1)  [unwired: 8 in, 1 out]
        "TMD37003 Data" <- w84
        n45 = call-poly <vilib>:"PwF_TMD37003_RGBToHSV.vi"("TMD37003 Data In"=w84) -> ("Hue"=w83:dbl)  [unwired: 3 out]
        n46 = Unbundle By Name(w80) -> ("status"=w76:bool)
        n47 = call "Hue_Color_value.vi"("Hue"=w83) -> ("Color"=→"Color":T2)
        n48 = First Call?() -> (First Call?: T/F=w77:bool)
        n49 = Compound Arithmetic op=AND(w76, invert w77) -> (w75:bool)
        n50 = call "Timed_DeBounce.vi"("Input"=w75, "Hold Time(ms)"=u32 5000) -> ("Output"=w78:bool)  [unwired: 1 in]
      }
      frame True {
      }
    }
    n51 = call "control_panel_manual.vi"("ManualCntrl_command"=w70, "MaualCntrlDevRef"=w69) -> ()  [unwired: 2 in]
    n52 = Wait (ms)(milliseconds to wait=u32 50) -> ()  [unwired: 1 out]
  }
  n53 = while {
    shift-right: [w89] -> _
    shift-left: w2 -> [w89]
    stop <- w87 stop-if-true
    # "Compressor"
    n54 = Unbundle By Name(w89) -> ("Pneumatics.Compressor"=w88:T37, "RobotConfig.EnableCompressor"=w86:bool)
    n55 = Not(x=w86) -> (.not. x?=w87:bool)
    n56 = case shown="True" w86 {
      tunnel: w88 -> [_ w91]
      frame False {
      }
      frame True {
        n57 = call <vilib>:"WPI_CompressorGetEnableState.vi"("CompressorDevRef"=w91) -> ()  [unwired: 7 in, 4 out]
      }
    }
    n58 = Wait (ms)(milliseconds to wait=u32 100) -> ()  [unwired: 1 out]
  }
  n59 = while {
    shift-right: [w131] -> _
    shift-left: w2 -> [w131]
    stop <- FALSE stop-if-true
    # "Shooter"
    n60 = Unbundle By Name(w131) -> ("RobotConfig.PID.Hood"=w148:T12, "RobotConfig.MotionLimits.Hood.Min (deg)"=w170:dbl, "RobotConfig.MotionLimits.Hood.Max (deg)"=w171:dbl, "MotorRefNumsOut.ShooterHood"=w174:T31, "RobotConfig.Motors.ShooterHood"=w175:T7, "RobotConfig.Homing.Hood Homing Position (deg)"=w176:dbl)
    n61 = Unbundle By Name(w131) -> ("RobotConfig.PID.Turret"=w136:T12, "RobotConfig.MotionLimits.Turret.Min (deg)"=w165:dbl, "RobotConfig.MotionLimits.Turret.Max (deg)"=w166:dbl, "MotorRefNumsOut.ShooterRotate"=w140:T31, "RobotConfig.Motors.ShooterRotate"=w138:T7, "RobotConfig.Homing.Turret Homing Position (deg)"=w164:dbl)
    n62 = global read "JoystickControls.vi" "JoystickControls"() -> (w179:T40)
    n63 = Unbundle By Name(w131) -> ("RobotConfig.CameraMounting.RotationRadius(in)"=w101:dbl, "RobotConfig.CameraMounting.LensHeight(in)"=w156:dbl, "RobotConfig.CameraMounting.Pitch(deg)"=w155:dbl)
    n64 = call <vilib>:"WPI_DriverStationOutputsEnabled.vi"() -> ("OutputsEnabled?"=w117:bool)  [unwired: 10 in, 1 out]
    n65 = global read "JoystickControls.vi" "JoystickControls"() -> (w161:T40)
    n66 = global read "JoystickControls.vi" "JoystickControls"() -> (w154:T40)
    n67 = Unbundle By Name(w179) -> ("H U/D"=w178:dbl)
    n68 = call "Shooter_Hood_Control_Manual.vi"("Hood_Command"=w178) -> ("ShooterHoodMotorCommand"=w177:dbl)
    n69 = feedback #1() -> (w118:T3)  [unwired: 1 in]
    n70 = call "Auto-Home_Startup.vi"("Enabled?"=w117, "Enum"=w118) -> ("Activate_Auto-Home"=w115:bool)
    n71 = Or(x="HoodHomeActivate", y=w115) -> (x .or. y?=w116:bool)
    n72 = Unbundle By Name(w161) -> ("H L/R"=w162:dbl)
    n73 = Unbundle By Name(w154) -> ("Find Target"=w121:bool)
    n74 = feedback #2() -> (w96:T42)  [unwired: 1 in]
    n75 = Unbundle By Name(w96) -> ("Valid"=w95:bool, "Angle(deg)"=w94:dbl, "FieldCentricAngle(deg)"=w93:dbl)
    n76 = call "Auto_Zoom_Limelight.vi"("Target_Horizontal Angle"=w93, "Verticle_Angle"=w94, "Is_Target_Visible?"=w95) -> ("Zoom_Indicator"=w92:T41)
    n77 = call "Shooter_Hood_Homing.vi"("Controller_Command"=w177, "Home_Position"=w176, "Homing Activated"=w116, "Reset"="HoodHomeReset", "Hood_Motor_DevRef"=w174, "MotorConfig"=w175) -> ("Homing_State"=w102:T3, "Motor_Output"=w173:dbl, "MotorConfig Out"=w147:T7, "Hood_Motor_DevRefOut"=w120:T31)
    "Hood_Homing_State" <- w102
    n78 = feedback-in #1(w102) -> ()
    n79 = call "Turret_Control_Manual.vi"("Rotate_Command"=w162) -> ("TurretMotorCommand"=w163:dbl)
    n80 = call "Turret_Homing.vi"("Controller_Command"=w163, "Turret_Motor_DefRef"=w140, "TurretManualHoming"="Turret Homing Activated", "Reset"="TurretHomeReset", "Home_Position"=w164, "MotorConfig"=w138) -> ("Motor_Output"=w167:dbl, "Homing_State"=w168:T3, "Turret_Motor_DefRef Out"=w139:T31, "MotorConfigOut"=w137:T7)  [unwired: 2 in]
    "Turret Homing_State" <- w168
    n81 = Select(t=w92, s=w121, f=VisionPipeline."LEDOff" ("pipeline control")) -> (s? t:f=w152:T41)
    n82 = call "VisionGetTarget.vi"("pipeline control"=w152, "Camera Pitch [deg.]"=w155, "Camera Height[in.]"=w156, "Limelight name"="limelight") -> ("VisionTarget"=w97:T42)  [unwired: 6 in, 1 out]
    n83 = feedback-in #2(w97) -> ()
    n84 = Equal?(x=w168, y=Hood_Homing_State."Homing in Process") -> (x = y?=w169:bool)
    n85 = Unbundle By Name(w131) -> ("RobotConfig.Motors.LeftShooter"=w98:T7, "MotorRefNumsOut.LeftShooter"=w135:T31, "MotorRefNumsOut.RightShooter"=w107:T31, "RobotConfig.PID.Shooter"=w109:T12)
    n86 = Unbundle By Name(w97) -> ("Valid"=w113:bool)  [unwired: 1 out]
    n87 = global read "JoystickControls.vi" "JoystickControls"() -> (w134:T40)
    n88 = call "limelight-turret_converter.vi"("VisionTarget"=w97, "Limelight Radius (in)"=w101) -> ("Turret Yaw Angle (deg)"=w99:dbl, "Turret Distance (in)"=w100:dbl)
    "Turret Distance (in)" <- w100
    n89 = Not(x="ManualShooterSpeed") -> (.not. x?=w106:bool)
    n90 = call "Target_Distances.vi"("Distance_to_target (in)"=w100) -> ("Shooter_RPM_Output"=w130:dbl, "Hood_Angle_Output (Deg)"=w114:dbl)
    n91 = Unbundle By Name(w97) -> ("Valid"=→"Target Found?":bool)
    n92 = Unbundle By Name(w134) -> ("Spin up"=w133:bool)
    n93 = feedback #3("ShooterSpeed(rpm)") -> (w104:dbl)
    n94 = Select(t=w130, s=w113, f=w104) -> (s? t:f=w105:dbl)
    n95 = feedback-in #3(w105) -> ()
    n96 = Select(t=w105, s=w106, f="ShooterSpeed(rpm)") -> (s? t:f=w111:dbl)
    n97 = Select(t=w111, s=w133, f=0.0) -> (s? t:f=w108:dbl)
    n98 = feedback #4() -> (w129:dbl)  [unwired: 1 in]
    n99 = feedback #5(TRUE ("Manual?")) -> (w143:bool)
    n100 = call "TurretSetpointSelect.vi"("TurretManualControlActive"=w143, "ManualSetpointEnable"="DisableLimelight", "CurrentTurretPosition(deg)"=w129, "ManualSetpointActivate"="Activate Auto (Turret)", "VisionTarget"=w97, "limelight_set_point"=w99, "AutoTargetActivate"=w121, "ManualSetpoint(deg)"="SetPointTurret(Deg)") -> ("Setpoint(deg)"=w144:dbl, "ActivateAutoControl"=w145:bool)  [unwired: 2 in]
    n101 = call "ShooterControl.vi"("MotorConfig"=w98, "PIDParams"=w109, "Setpoint (rpm)"=w108, "FollowerMotorControlDevRef"=w107, "LeaderMotorControlDevRef"=w135) -> ("Sensor Velocity"=→"Shooter Velocity":dbl)  [unwired: 4 in]
    n102 = call "TurretAngleControl.vi"("TurretMotorControlDevRef"=w139, "Activate Auto"=w145, "MaxDegrees"=w166, "Homing"=w169, "MinDegrees"=w165, "MotorConfig"=w137, "SetPoint(Deg)"=w144, "ManualControl"=w167, "PIDParams"=w136) -> ("Manual?"=w150:bool, "Current Position (Deg)"=w151:dbl)  [unwired: 5 in]
    "Turret Current Position (Deg)" <- w151
    "TurretManual" <- w150
    n103 = feedback-in #4(w151) -> ()
    n104 = feedback-in #5(w150) -> ()
    n105 = feedback #6(TRUE ("Manual?")) -> (w123:bool)
    n106 = call "HoodSetpointSelect.vi"("HoodManualControlActive"=w123, "ManualSetpointEnable"="DisableLimelight", "ManualSetpointActivate"="Activate Auto (Shooter Hood)", "VisionTarget"=w97, "HoodAutoAimAngle"=w114, "AutoTargetActivate"=w121, "ManualSetpoint(deg)"="SetPointHood(Deg)") -> ("Setpoint(deg)"=w119:dbl, "ActivateAutoControl"=w122:bool)  [unwired: 3 in]
    n107 = call "ShooterHoodPositionControl.vi"("ShooterHoodMotorControlDevRef"=w120, "Activate Auto"=w122, "MaxDegrees"=w171, "HoodHomingState"=w102, "MinDegrees"=w170, "MotorConfig"=w147, "SetPoint(Deg)"=w119, "ManualControl"=w173, "PIDParams"=w148) -> ("Manual?"=w125:bool, "Current Position (Deg)"=→"Hood Current Position (Deg)":dbl)  [unwired: 3 in, 2 out]
    "HoodManual?" <- w125
    n108 = feedback-in #6(w125) -> ()
    n109 = Wait (ms)(milliseconds to wait=u32 20) -> ()  [unwired: 1 out]
  }
